vi "IniProcess.vi"(7 "操作模式":T1, 8 "error in (no error)":errorcluster caption="错误输入（无错误）", 9 "Ctls":refnum<vi>[](array[refnum]), 10 "section":string caption="段", 11 "configuration file path":path caption="配置文件的路径") -> (0 "error out":errorcluster caption="错误输出", 3 "配置文件":path)   [LabVIEW 2012, in "IniReader&WriterForControl.lvlib"]
uses:
  IniReader&WriterForControl.lvlib
  ProcessMode.ctl
  <vilib>/Utility/config.llb/NI_LVConfig.lvlib
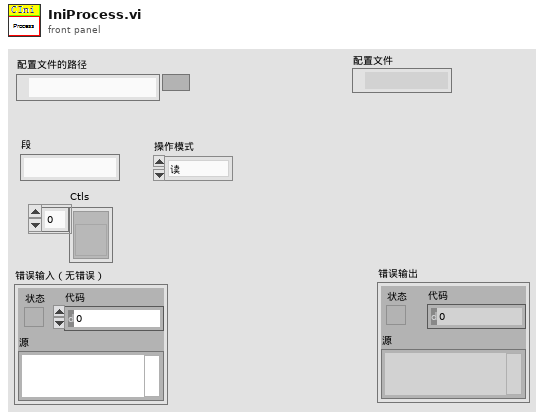
[diagram p1: front panel]
types:
  T1 = typedef "IniReader&WriterForControl.lvlib/ProcessMode.ctl" = enum16{"读", "写"}
  T2 = typedef "NI_LVConfig.lvlib/Config Data RefNum.ctl" = refnum<k1>
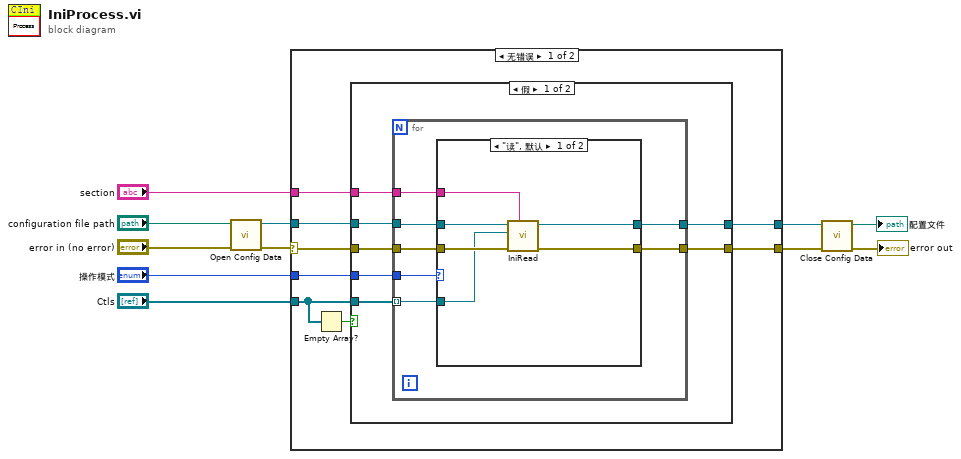
[diagram p0: block diagram]
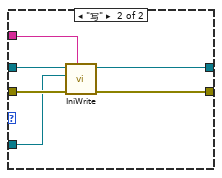
[diagram p2: hidden frame]
diagram:
  n1 = call <vilib>:"Open Config Data.vi"("error in (no error)"="error in (no error)", "configuration file path"="configuration file path") -> ("error out"=w8:errorcluster, "refnum"=w9:T2)  [unwired: 7 in, 1 out]
  n2 = case shown="无错误" w8 {
    selector: w8 -> [w18 w48]
    tunnel: "Ctls" -> [w17 _]
    tunnel: w9 -> [w19 w49]
    tunnel: "操作模式" -> [w15 _]
    tunnel: "section" -> [w14 _]
    tunnel: [w13 w48] -> w5
    tunnel: [w12 w49] -> w4
    frame No Error {
      n3 = Empty Array?(array=w17) -> (empty?=w16:bool)
      n4 = case shown="假" w16 {
        tunnel: w19 -> [w26 w47]
        tunnel: w18 -> [w25 w46]
        tunnel: w17 -> [w24 _]
        tunnel: w15 -> [w23 _]
        tunnel: w14 -> [w22 _]
        tunnel: [w21 w46] -> w13
        tunnel: [w20 w47] -> w12
        frame False {
          n5 = for {
            tunnel: w26 -> [w31]
            tunnel: w25 -> [w32]
            tunnel: w24 -> [w30] mode=indexing
            tunnel: w23 -> [w33]
            tunnel: w22 -> [w29]
            tunnel: [w28] -> w20
            tunnel: [w27] -> w21
            n6 = case shown="\"读\", 默认" w33 {
              tunnel: w32 -> [w39 w45]
              tunnel: w31 -> [w38 w44]
              tunnel: w30 -> [w37 w43]
              tunnel: w29 -> [w36 w42]
              tunnel: [w35 w41] -> w28
              tunnel: [w34 w40] -> w27
              frame "读", Default {
                n7 = call "IniRead.vi"("section"=w36, "error in (no error)"=w39, "控件引用"=w37, "Ini.In"=w38) -> ("error out"=w34:errorcluster, "Ini.Out"=w35:T2)  [unwired: 6 in]
              }
              frame "写" {
                n8 = call "IniWrite.vi"("section"=w42, "error in (no error)"=w45, "控件引用"=w43, "Ini.In"=w44) -> ("error out"=w40:errorcluster, "Ini.Out"=w41:T2)  [unwired: 6 in]
              }
            }
          }
        }
        frame True {
        }
      }
    }
    frame Error {
    }
  }
  n9 = call <vilib>:"Close Config Data.vi"("error in (no error)"=w5, "refnum"=w4) -> ("error out"=→"error out":errorcluster, "file path"=→"配置文件":path)  [unwired: 8 in]
